vi "2. Cast Image.vi"() -> ()   [LabVIEW 2019]
doc: "c 2020 ReMiSYS All rights reserved."
panel:
  in  "All Images? (No)":bool
  in  "Image Type":T1 items=["Grayscale (U8)", "Grayscale (I16)", "Grayscale (SGL)", "Complex (CSG)", "RGB (U32)", "HSL (U32)", "RGB (U64)", "Grayscale (U16)"]
  out "Gray Image":T2(plugin-control)
  in  "Stop (F)":bool
  out "Ori Image":T2(plugin-control)
  # "IMAQ Dispose  (Dispose All Images?)"
  # "c 2022 ReMiSYS All rights reserved."
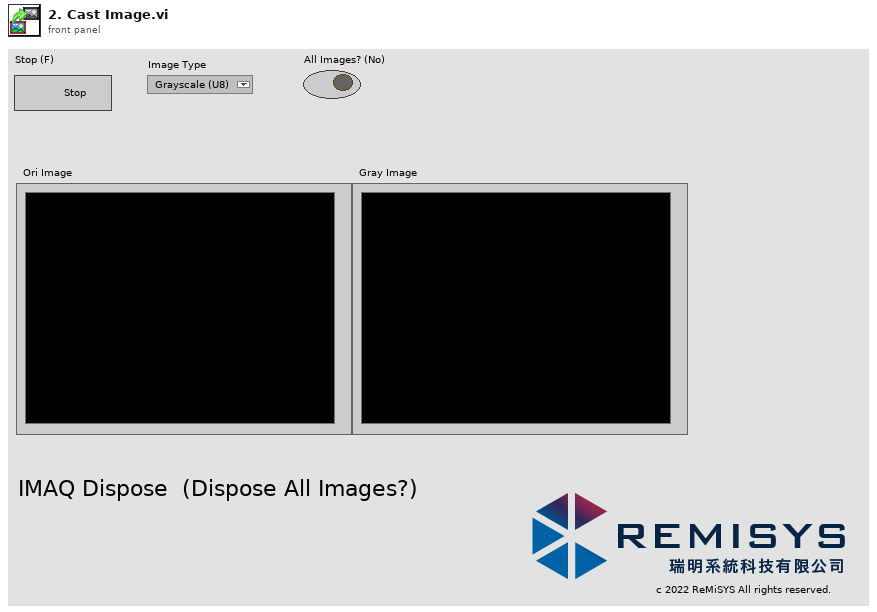
[diagram p1: front panel]
types:
  T1 = typedef "Image Type" = u32
  T2 = typedef "IMAQ Image.ctl" = refnum<image>
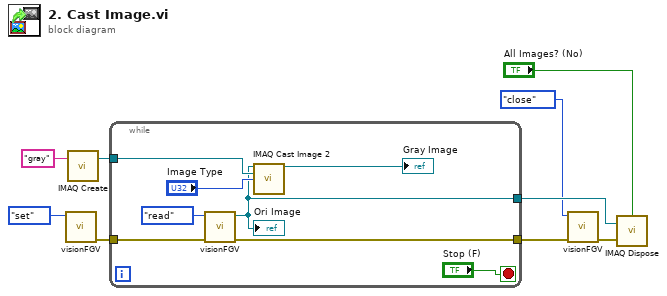
[diagram p0: block diagram]
diagram:
  n1 = call "visionFGV.vi"("Function"=enum16{"set", "read", "close"}."set") -> ("error out"=w5:errorcluster)  [unwired: 9 in, 1 out]
  n2 = call "IMAQ Create"("Image Name"="gray") -> ("New Image"=w7:T2)  [unwired: 4 in, 1 out]
  n3 = while {
    tunnel: [w12] -> w9
    tunnel: w7 -> [w17]
    tunnel: w5 -> [w13]
    tunnel: [w10] -> w3
    stop <- "Stop (F)" stop-if-true
    n4 = call "visionFGV.vi"("Error In"=w13, "Function"=enum16{"set", "read", "close"}."read") -> ("error out"=w10:errorcluster, "Image Out fgv"=w12:T2)  [unwired: 8 in]
    "Ori Image" <- w12
    n5 = call "IMAQ Cast Image 2"("Image Src"=w12, "Image Dst"=w17, "Image Type"="Image Type") -> ("Image Dst Out"=→"Gray Image":T2)  [unwired: 11 in, 1 out]
  }
  n6 = call "visionFGV.vi"("Error In"=w3, "Function"=enum16{"set", "read", "close"}."close") -> ("error out"=w2:errorcluster)  [unwired: 8 in, 1 out]
  n7 = call "IMAQ Dispose"("All Images? (No)"="All Images? (No)", "Image"=w9, "error in (no error)"=w2) -> ()  [unwired: 3 in, 1 out]
